vi "testing_queues.vi"() -> ()   [LabVIEW 2015]
panel:
  out "Numeric 2":i32
  in  "stop 2":bool
  in  "stop":bool
  out "element":i32
  out "Numeric":i32
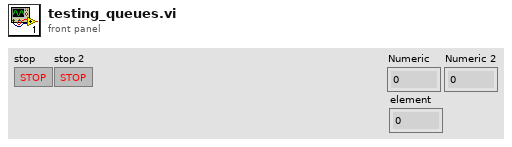
[diagram p1: front panel]
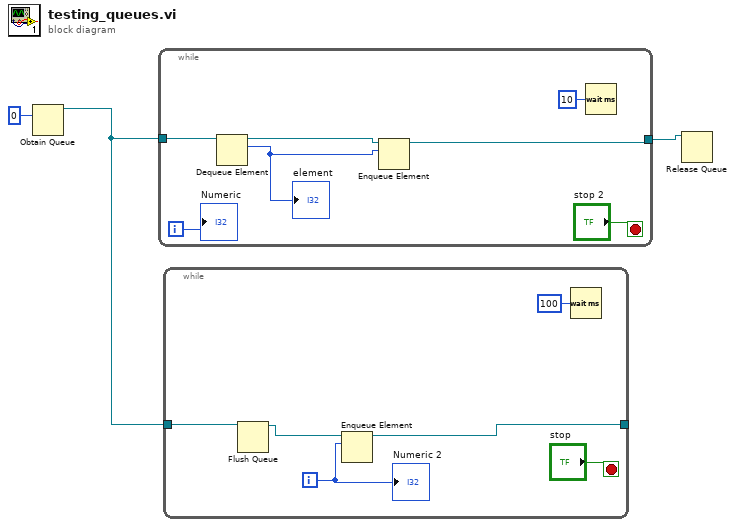
[diagram p0: block diagram]
diagram:
  n1 = Obtain Queue(element data type=0) -> (queue out=w2:refnum<queue>)  [unwired: 4 in, 2 out]
  n2 = while {
    tunnel: w2 -> [w9]
    tunnel: [w4] -> w1
    i -> [w8]
    stop <- "stop 2" stop-if-true
    n3 = Dequeue Element(queue=w9) -> (queue out=w6:refnum<queue>, element=w5:i32)  [unwired: 2 in, 2 out]
    "element" <- w5
    n4 = Enqueue Element(queue=w6, element=w5) -> (queue out=w4:refnum<queue>)  [unwired: 2 in, 2 out]
    n5 = Wait (ms)(milliseconds to wait=u32 10) -> ()  [unwired: 1 out]
    "Numeric" <- w8
  }
  n6 = while {
    tunnel: w2 -> [w12]
    tunnel: [w13] -> _
    i -> [w15]
    stop <- "stop" stop-if-true
    n7 = Flush Queue(queue=w12) -> (queue out=w11:refnum<queue>)  [unwired: 1 in, 2 out]
    n8 = Enqueue Element(queue=w11, element=w15) -> (queue out=w13:refnum<queue>)  [unwired: 2 in, 2 out]
    n9 = Wait (ms)(milliseconds to wait=u32 100) -> ()  [unwired: 1 out]
    "Numeric 2" <- w15
  }
  n10 = Release Queue(queue=w1) -> ()  [unwired: 2 in, 3 out]
